vi "Tester.vi"() -> ()   [LabVIEW 2018, in "E-Series Reader.lvlib"]
uses:
  E-Series Reader.lvlib
  Series Data--cluster.ctl
panel:
  in  "INI File":string="e-series files names.ini"
  out "Series Data":T1
  # "Tester for \nLoad E-Series VI"
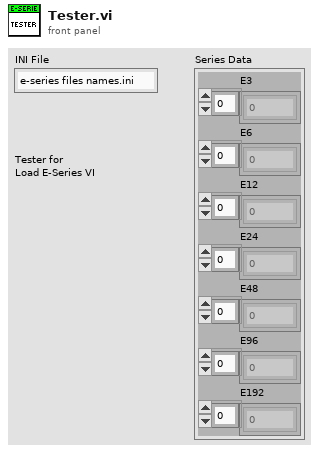
[diagram p1: front panel]
types:
  T1 = typedef "E-Series Reader.lvlib/Series Data--cluster.ctl" = cluster{"E3":u16[], "E6":u16[], "E12":u16[], "E24":u16[], "E48":u16[], "E96":u16[], "E192":u16[]}
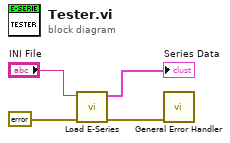
[diagram p0: block diagram]
diagram:
  n1 = call "Load E-Series.vi"("error in (no error)"=errorcluster {"status"=FALSE, "code"=0, "source"=""} ("error in"), "INI File"="INI File") -> ("error out"=w3:errorcluster, "E-Series Data"=→"Series Data":T1)  [unwired: 8 in]
  n2 = call <vilib>:"General Error Handler.vi"("error in (no error)"=w3) -> ()  [unwired: 10 in, 5 out]
